vi "Execute default event by ID.vi"(6 "Event Name":string, 8 "Module ID":i32, 9 "Module type":T1, 10 "Module Lib":refnum<vi>, 11 "References Map":map{string, refnum<vi>}(c390)) -> (0 "error out":errorcluster)   [LabVIEW 2019, in "Panther Dashboard.lvlib"]
uses:
  Panther Dashboard.lvlib
  Module type--enum.ctl
panel:
  out "Error Cleared?":bool
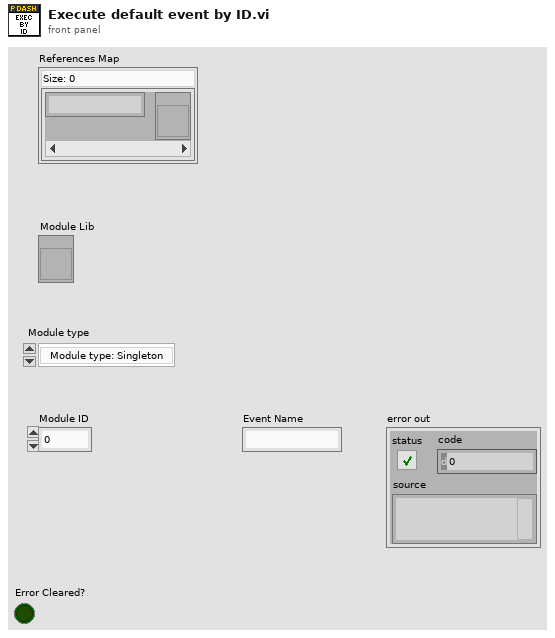
[diagram p1: front panel]
types:
  T1 = typedef "Panther Dashboard.lvlib/Module type--enum.ctl" = enum16{"Module type: Singleton", "Module type: Cloneable"}
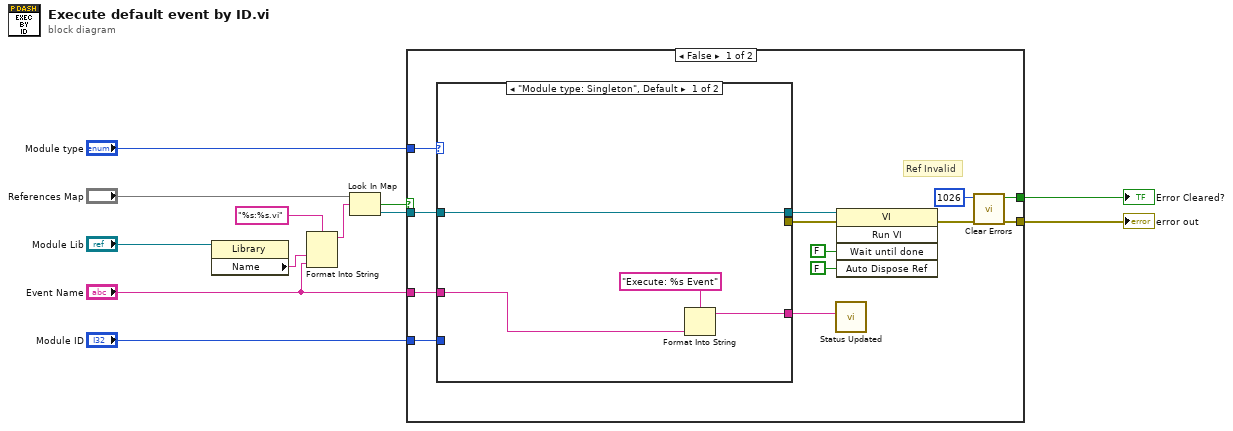
[diagram p0: block diagram]
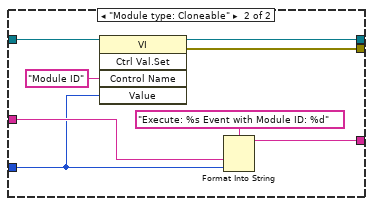
[diagram p2: hidden frame]
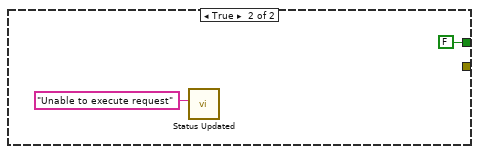
[diagram p3: hidden frame]
diagram:
  n1 = property class="Library"(reference="Module Lib") -> ("Name"=w6:string)  [unwired: 1 in, 2 out]
  n2 = Format Into String(format string="%s:%s.vi", w6, "Event Name") -> (resulting string=w11:string)  [unwired: 2 in, 1 out]
  n3 = Look In Map(map="References Map", key=w11) -> (key not found?=w3:bool, value=w9:refnum<vi>)  [unwired: 1 in]
  n4 = case shown="False" w3 {
    tunnel: w9 -> [w22 _]
    tunnel: "Module ID" -> [w21 _]
    tunnel: "Module type" -> [w19 _]
    tunnel: "Event Name" -> [w18 _]
    tunnel: [w14 _] -> w2
    tunnel: [w13 FALSE ("specific error cleared?")] -> w1
    frame False {
      # "Ref Invalid"
      n5 = case shown="\"Module type: Singleton\", Default" w19 {
        tunnel: [_ w37] -> w25
        tunnel: w22 -> [w29 w36]
        tunnel: w21 -> [_ w32]
        tunnel: [w29 w34] -> w20
        tunnel: w18 -> [w28 w33]
        tunnel: [w27 w31] -> w17
        frame "Module type: Singleton", Default {
          n6 = Format Into String(format string="Execute: %s Event", w28) -> (resulting string=w27:string)  [unwired: 2 in, 1 out]
        }
        frame "Module type: Cloneable" {
          n7 = invoke class="VI" method="Ctrl Val.Set"(reference=w36, "Control Name"="Module ID", "Value"=w32) -> (reference out=w34:refnum<vi>, error out=w37:errorcluster)  [unwired: 2 in, 3 out]
          n8 = Format Into String(format string="Execute: %s Event with Module ID: %d", w33, w32) -> (resulting string=w31:string)  [unwired: 2 in, 1 out]
        }
      }
      n9 = call "Status Updated.vi"("Status"=w17) -> ()  [unwired: 10 in, 1 out]
      n10 = invoke class="VI" method="Run VI"(reference=w20, error in=w25, "Wait until done"=FALSE ("Wait Until Done"), "Auto Dispose Ref"=FALSE ("Auto Dispose Reference")) -> (error out=w16:errorcluster)  [unwired: 1 in, 4 out]
      n11 = call <vilib>:"Clear Errors.vi"("error in (no error)"=w16, "specific error code to clear (0: all)"=1026) -> ("error out"=w14:errorcluster, "specific error cleared?"=w13:bool)  [unwired: 4 in]
    }
    frame True {
      n12 = call "Status Updated.vi"("Status"="Unable to execute request") -> ()  [unwired: 10 in, 1 out]
    }
  }
  "error out" <- w2
  "Error Cleared?" <- w1
